vi "Get NumOfImages.vi"(8 "error in (no error)":errorcluster, 11 "ImageOperation in":refnum<class "ImageOperation.lvclass">) -> (0 "error out":errorcluster, 2 "NumOfImages":i32, 3 "ImageOperation out":refnum<class "ImageOperation.lvclass">)   [LabVIEW 2015, in "ImageOperation.lvclass"]
uses:
  ImageOperation.lvclass
  ImageOperation.lvclass/ImageOperation.ctl
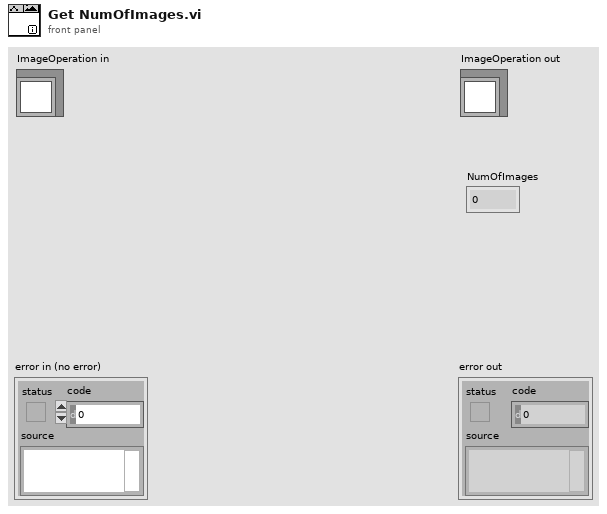
[diagram p1: front panel]
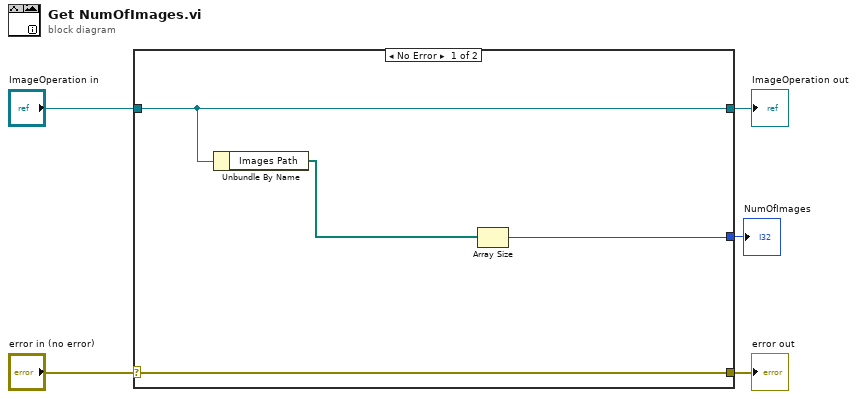
[diagram p0: block diagram]
diagram:
  n1 = case shown="No Error" "error in (no error)" {
    selector: "error in (no error)" -> [w9 w11]
    tunnel: [w9 w11] -> w4
    tunnel: [w8 w10] -> w2
    tunnel: "ImageOperation in" -> [w8 w10]
    tunnel: [w6 _] -> w1
    frame No Error {
      n2 = Unbundle By Name(w8) -> ("Images Path"=w7:path[])
      n3 = Array Size(array=w7) -> (size(s)=w6:i32)
    }
    frame Error {
    }
  }
  "error out" <- w4
  "ImageOperation out" <- w2
  "NumOfImages" <- w1
